vi "Pre Launch Init.vi"(11 "CS++ObjectManager in":refnum<class "CS++ObjectManager.lvclass">) -> (0 "Error Out":errorcluster, 3 "CS++ObjectManager out":refnum<class "CS++ObjectManager.lvclass">)   [LabVIEW 2015, in "CS++ObjectManager.lvlib" / "CS++ObjectManager.lvclass"]
doc: "Create GUI Events.\n\n(<B>Filename</B>: Actor Framework.lvlib:Actor.lvclass:Pre Launch Init.vi)\n\nDefines behavior that occurs after the Launch Actor method is invoked but before the actor's Actor Core method begins running.\n\nThe Pre Launch Init method is guaranteed to finish before the Launch Actor method returns to its caller and before the actor itself receives any messages. Any references that the Pre Launch Init method obtains are guaranteed to have the same lifetime as the actor itself. Any errors that the Pre Launch Init method returns will abort the launch.\n\nBy default, this method does nothing. A descendant class may override it to define behavior."
uses:
  CS++ObjectManager.lvclass
  <vilib>/ActorFramework/Message Enqueuer/Message Enqueuer.lvclass
  CS++ObjectManager.lvclass/CS++ObjectManager.ctl
  CSPP_Core/Actors/CS++GUIActor/CS++GUIActor.lvclass
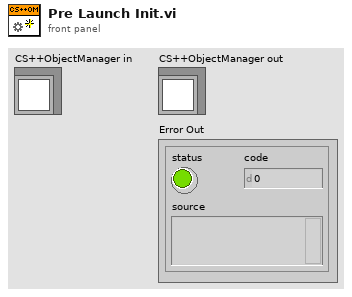
[diagram p1: front panel]
types:
  T1 = cluster{"Actor Names":string[], "Actor Class & Enqueuer":cluster{"Class Name":string, "Enqueuer":refnum<class "Message Enqueuer.lvclass">}[]}
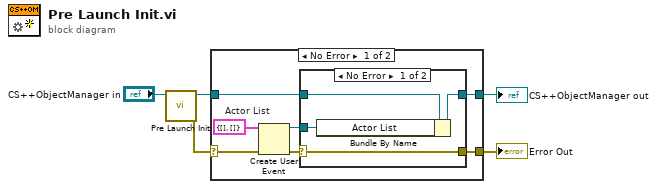
[diagram p0: block diagram]
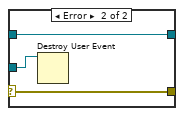
[diagram p2: hidden frame]
diagram:
  n1 = call-parent "Pre Launch Init.vi"("CS++GUIActor in"="CS++ObjectManager in") -> ("error out"=w3:errorcluster, "CS++GUIActor out"=w4:refnum<class "CS++ObjectManager.lvclass">)  [unwired: 9 in]
  n2 = case shown="No Error" w3 {
    selector: w3 -> [w12 w20]
    tunnel: w4 -> [w11 w21]
    tunnel: [w10 w21] -> w2
    tunnel: [w9 w20] -> w1
    frame No Error {
      w6 = T1 {"Actor Names"=[], "Actor Class & Enqueuer"=[]}  # Actor List
      n3 = Create User Event(user event datatype=w6, error in=w12) -> (user event=w8:refnum<user-event>, error out=w7:errorcluster)
      n4 = case shown="No Error" w7 {
        selector: w7 -> [w14 w17]
        tunnel: w8 -> [w13 w19]
        tunnel: w11 -> [w16 w18]
        tunnel: [w15 w18] -> w10
        tunnel: [w14 w17] -> w9
        frame No Error {
          n5 = Bundle By Name(cluster=w16, "Actor List"=w13) -> (w15:refnum<class "CS++ObjectManager.lvclass">)
        }
        frame Error {
          n6 = Destroy User Event(user event=w19) -> ()  [unwired: 1 in, 1 out]
        }
      }
    }
    frame Error {
    }
  }
  "Error Out" <- w1
  "CS++ObjectManager out" <- w2
